vi "make_log_file_H5.vi"(0 "Path":path, 1 "Log Cluster":T2, 2 "Flow Data":T1) -> ()   [LabVIEW 2016]
uses:
  <vilib>/addons/h5labview2/file/H5Fmode.ctl
  <vilib>/addons/h5labview2/base/lib_path.vi
  <vilib>/addons/h5labview2/base/H5Equery.vi
  <vilib>/addons/h5labview2/dataset/H5Dwrite.llb/H5Dwrite.xnode
  <vilib>/addons/h5labview2/file/H5F.lvlib
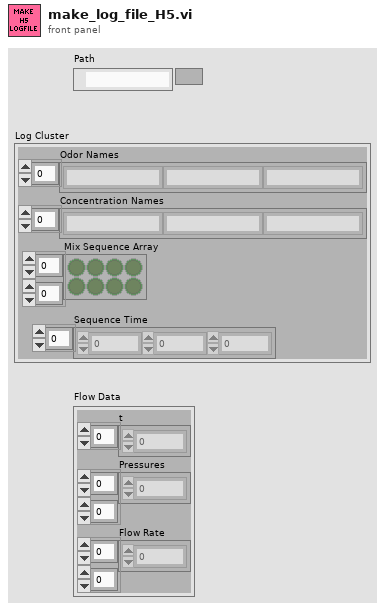
[diagram p1: front panel]
types:
  T1 = cluster{"t":dbl[], "Pressures":dbl[][], "Flow Rate":dbl[][]}
  T2 = cluster{"Odor Names":string[], "Concentration Names":string[], "Mix Sequence Array":bool[][], "Sequence Time":dbl[]}
  T3 = typedef "H5F.lvlib/H5Fmode.ctl" = enum16{"read-only", "read-write", "overwrite", "create new", "open or create"}
  T4 = typedef "hid_t.ctl" = i32
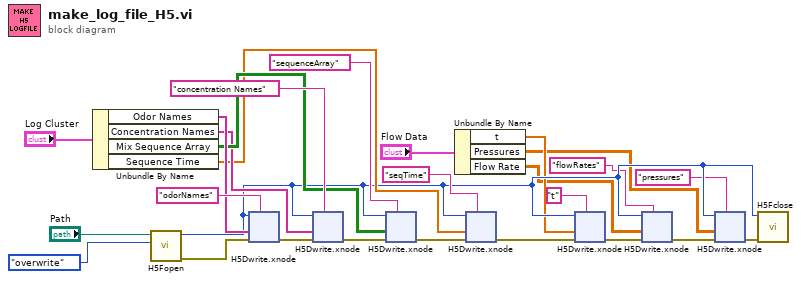
[diagram p0: block diagram]
diagram:
  n1 = Unbundle By Name("Log Cluster") -> ("Odor Names"=w22:string[], "Concentration Names"=w18:string[], "Mix Sequence Array"=w19:bool[][], "Sequence Time"=w13:dbl[])
  n2 = call <vilib>:"H5Fopen.vi"("mode (read-only)"=H5Fmode."overwrite", "path"="Path") -> ("error out"=w24:errorcluster, "ref out"=w11:T4)  [unwired: 8 in]
  n3 = xnode "H5Dwrite.xnode"("dataset name"="odorNames", "error in (no error)"=w24, "data"=w22, "ref in"=w11) -> ("error out"=w17:errorcluster)  [unwired: 3 in, 2 out]
  n4 = xnode "H5Dwrite.xnode"("dataset name"="concentration Names", "error in (no error)"=w17, "data"=w18, "ref in"=w11) -> ("error out"=w16:errorcluster)  [unwired: 3 in, 2 out]
  n5 = xnode "H5Dwrite.xnode"("dataset name"="sequenceArray", "error in (no error)"=w16, "data"=w19, "ref in"=w11) -> ("error out"=w15:errorcluster)  [unwired: 3 in, 2 out]
  n6 = Unbundle By Name("Flow Data") -> ("t"=w3:dbl[], "Pressures"=w1:dbl[][], "Flow Rate"=w2:dbl[][])
  n7 = xnode "H5Dwrite.xnode"("dataset name"="seqTime", "error in (no error)"=w15, "data"=w13, "ref in"=w11) -> ("error out"=w10:errorcluster)  [unwired: 3 in, 2 out]
  n8 = xnode "H5Dwrite.xnode"("dataset name"="t", "error in (no error)"=w10, "data"=w3, "ref in"=w11) -> ("error out"=w9:errorcluster)  [unwired: 3 in, 2 out]
  n9 = xnode "H5Dwrite.xnode"("dataset name"="flowRates", "error in (no error)"=w9, "data"=w2, "ref in"=w11) -> ("error out"=w8:errorcluster)  [unwired: 3 in, 2 out]
  n10 = xnode "H5Dwrite.xnode"("dataset name"="pressures", "error in (no error)"=w8, "data"=w1, "ref in"=w11) -> ("error out"=w7:errorcluster)  [unwired: 3 in, 2 out]
  n11 = call <vilib>:"H5Fclose.vi"("error in (no error)"=w7, "ref"=w11) -> ()  [unwired: 9 in, 1 out]
